vi "Get Hardware Status.vi"(4 "error in (no error)":errorcluster, 7 "VISA resource name":refnum<visa-resource-name>) -> (0 "error out":errorcluster, 1 "Status register 2":T1, 2 "Status register 1":T2, 3 "VISA resource name out":refnum<visa-resource-name>)   [LabVIEW 2010, in "Newport ESP301.lvlib"]
doc: "Reads hardware status for all axis."
uses:
  <userlib>/Newport ESP301/Newport ESP301.lvlib
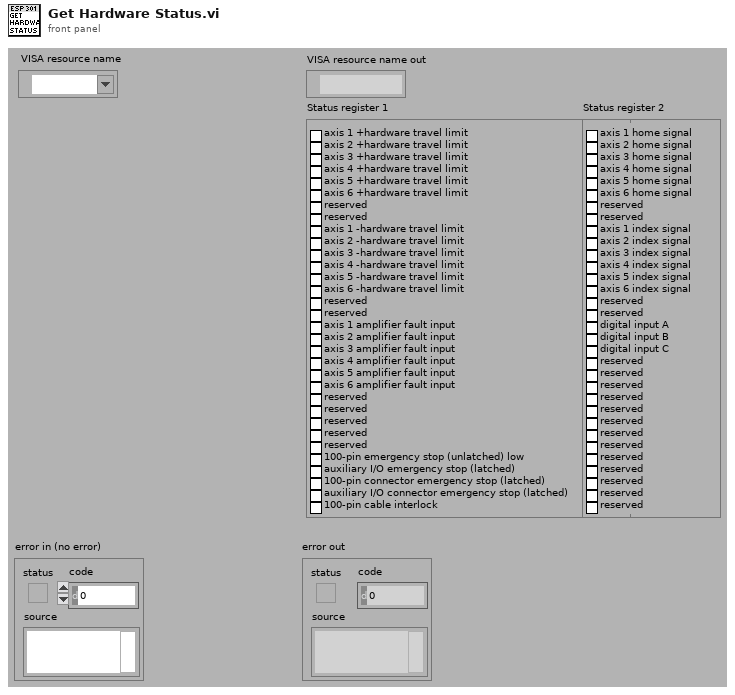
[diagram p1: front panel]
types:
  T1 = cluster{"axis 1 home signal":bool, "axis 2 home signal ":bool, "axis 3 home signal ":bool, "axis 4 home signal":bool, "axis 5 home signal":bool, "axis 6 home signal":bool, "reserved":bool, "reserved":bool, "axis 1 index signal":bool, "axis 2 index signal":bool, "axis 3 index signal":bool, "axis 4 index signal":bool, "axis 5 index signal":bool, "axis 6 index signal":bool, "reserved":bool, "reserved":bool, "digital input A":bool, "digital input B":bool, "digital input C":bool, "reserved":bool, "reserved":bool, "reserved":bool, "reserved":bool, "reserved":bool, "reserved":bool, "reserved":bool, "reserved":bool, "reserved":bool, "reserved":bool, "reserved":bool, "reserved":bool, "reserved":bool}
  T2 = cluster{"axis 1 +hardware travel limit":bool, "axis 2 +hardware travel limit ":bool, "axis 3 +hardware travel limit ":bool, "axis 4 +hardware travel limit ":bool, "axis 5 +hardware travel limit ":bool, "axis 6 +hardware travel limit ":bool, "reserved":bool, "reserved":bool, "axis 1 -hardware travel limit ":bool, "axis 2 -hardware travel limit ":bool, "axis 3 -hardware travel limit ":bool, "axis 4 -hardware travel limit ":bool, "axis 5 -hardware travel limit ":bool, "axis 6 -hardware travel limit ":bool, "reserved":bool, "reserved":bool, "axis 1 amplifier fault input":bool, "axis 2 amplifier fault input":bool, "axis 3 amplifier fault input":bool, "axis 4 amplifier fault input":bool, "axis 5 amplifier fault input":bool, "axis 6 amplifier fault input":bool, "reserved":bool, "reserved":bool, "reserved":bool, "reserved":bool, "reserved":bool, "100-pin emergency stop (unlatched) low":bool, "auxiliary I/O emergency stop (latched)":bool, "100-pin connector emergency stop (latched)":bool, "auxiliary I/O connector emergency stop (latched)":bool, "100-pin cable interlock":bool}
  T3 = cluster{"Boolean array[0]":bool, "Boolean array[1]":bool, "Boolean array[2]":bool, "Boolean array[3]":bool, "Boolean array[4]":bool, "Boolean array[5]":bool, "Boolean array[6]":bool, "Boolean array[7]":bool, "Boolean array[8]":bool, "Boolean array[9]":bool, "Boolean array[10]":bool, "Boolean array[11]":bool, "Boolean array[12]":bool, "Boolean array[13]":bool, "Boolean array[14]":bool, "Boolean array[15]":bool, "Boolean array[16]":bool, "Boolean array[17]":bool, "Boolean array[18]":bool, "Boolean array[19]":bool, "Boolean array[20]":bool, "Boolean array[21]":bool, "Boolean array[22]":bool, "Boolean array[23]":bool, "Boolean array[24]":bool, "Boolean array[25]":bool, "Boolean array[26]":bool, "Boolean array[27]":bool, "Boolean array[28]":bool, "Boolean array[29]":bool, "Boolean array[30]":bool, "Boolean array[31]":bool}
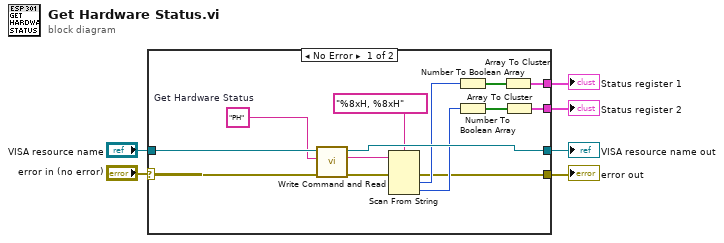
[diagram p0: block diagram]
diagram:
  n1 = case shown="No Error" "error in (no error)" {
    selector: "error in (no error)" -> [w18 w22]
    tunnel: [w7 w22] -> w6
    tunnel: "VISA resource name" -> [w20 w21]
    tunnel: [w19 w21] -> w5
    tunnel: [w10 _] -> w2
    tunnel: [w9 _] -> w1
    frame No Error {
      w17 = "PH"  # Get Hardware Status
      n2 = call <userlib>:"Write Command and Read.vi"("error in (no error)"=w18, "Command"=w17, "VISA resource name"=w20) -> ("error out"=w8:errorcluster, "Returned string"=w16:string, "VISA resource name out"=w19:refnum<visa-resource-name>)  [unwired: 2 in, 2 out]
      n3 = Scan From String(format string="%8xH, %8xH" ("chaîne de format"), input string=w16, error in=w8) -> (error out=w7:errorcluster, output 1=w14:i32, output 2=w13:i32)  [unwired: 3 in, 2 out]
      n4 = Number To Boolean Array(number=w14) -> (Boolean array=w12:bool[])
      n5 = Number To Boolean Array(number=w13) -> (Boolean array=w11:bool[])
      n6 = Array To Cluster(array=w12) -> (cluster=w10:T3)
      n7 = Array To Cluster(array=w11) -> (cluster=w9:T3)
    }
    frame Error {
    }
  }
  "error out" <- w6
  "VISA resource name out" <- w5
  "Status register 1" <- w2
  "Status register 2" <- w1
